vi "BasePath.vi"() -> (15 "BasePath":path)   [LabVIEW 2017]
doc: "Returns the path to the first two folders of the path to this vi."
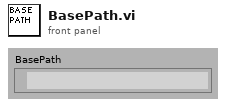
[diagram p1: front panel]
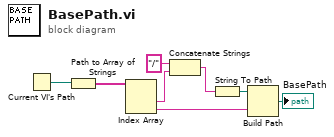
[diagram p0: block diagram]
diagram:
  n1 = Current VI's Path() -> (path=w1:path)
  n2 = Path to Array of Strings(0:w1) -> (2:w8:string[])  [unwired: 1 out]
  n3 = Index Array(array=w8) -> (element #1=w4:string, element #2=w6:string)  [unwired: 2 in]
  n4 = Concatenate Strings("/" ("string"), w4) -> (w2:string)
  n5 = String To Path(string=w2) -> (path=w7:path)
  n6 = Build Path(base path=w7, name or relative path=w6) -> (appended path=→"BasePath":path)
